vi "Send Message.vi"(8 "error in (no error)":errorcluster, 10 "Message":string, 11 "VISA Instrument in":refnum<class "VISA Instrument.lvclass">) -> (0 "error out":errorcluster, 3 "VISA Instrument out":refnum<class "VISA Instrument.lvclass">)   [LabVIEW 2020, in "VISA Instrument.lvclass"]
uses:
  VISA Instrument.lvclass
  VISA Instrument.lvclass/VISA Instrument.ctl
  Read VISA resource.vi
  Write VISA resource.vi
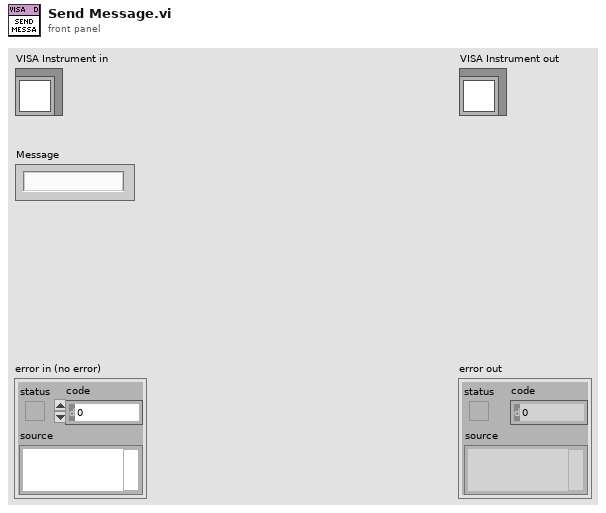
[diagram p1: front panel]
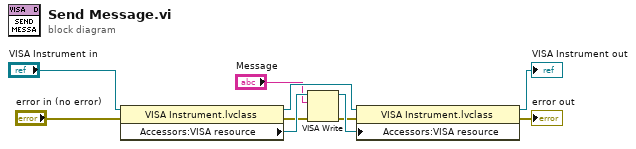
[diagram p0: block diagram]
diagram:
  n1 = property class="VISA Instrument.lvclass"(reference="VISA Instrument in", error in="error in (no error)") -> (reference out=w10:refnum<class "VISA Instrument.lvclass">, error out=w2:errorcluster, "Accessors:VISA resource"=w5:refnum<visa-resource-name>)
  n2 = VISA Write(VISA resource name=w5, write buffer="Message", error in (no error)=w2) -> (VISA resource name out=w4:refnum<visa-resource-name>, error out=w3:errorcluster)  [unwired: 1 out]
  n3 = property class="VISA Instrument.lvclass"(reference=w10, error in=w3, "Accessors:VISA resource"=w4) -> (reference out=→"VISA Instrument out":refnum<class "VISA Instrument.lvclass">, error out=→"error out":errorcluster)
